vi "Get Scaled FP to PicBox.vi"(7 "仅可见区域":bool, 8 "错误输入（无错误）":errorcluster, 10 "图像参数":cluster{"图像深度":i32, "最大宽度":i32, "最大高度":i32}={"图像深度"=8, "最大宽度"=0, "最大高度"=0} {"图像深度" items=["1位、黑白"=1, "4位、16色"=4, "8位、256色"=8, "24位、真彩色"=24]}, 11 "VI Ref":refnum<vi>) -> (0 "错误输出":errorcluster, 3 "二维图片":picture)   [LabVIEW 2012, in "VIRef.lvlib"]
uses:
  VIRef.lvlib
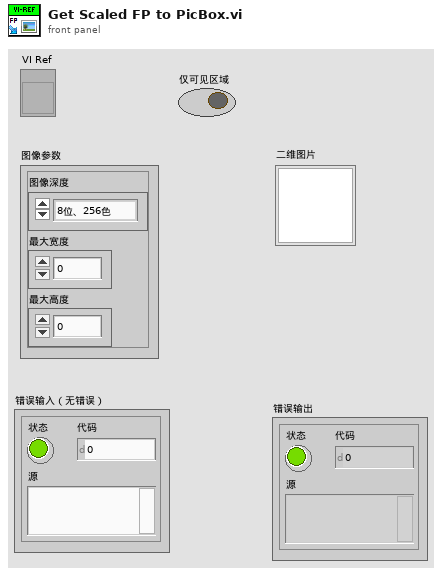
[diagram p1: front panel]
types:
  T1 = typedef "imagedata.ctl" = cluster{"image type":i32, "image depth":i32, "image":u8[], "mask":u8[], "colors":u32[], "Rectangle":cluster{"left":i16, "top":i16, "right":i16, "bottom":i16}}
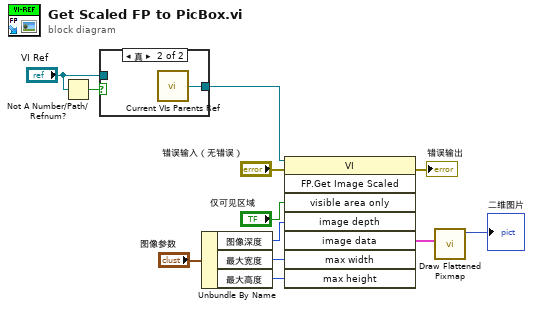
[diagram p0: block diagram]
diagram:
  n1 = Not A Number/Path/Refnum?(number/path/refnum="VI Ref") -> (NaN/Path/Refnum?=w12:bool)
  n2 = case shown="真" w12 {
    tunnel: [w13 w14] -> w10
    tunnel: "VI Ref" -> [w13 _]
    frame False {
    }
    frame True {
      n3 = call "Current VIs Parents Ref.vi"() -> ("Calling VI's Reference"=w14:refnum<vi>)  [unwired: 2 in]
    }
  }
  n4 = Unbundle By Name("图像参数") -> ("图像深度"=w7:i32, "最大宽度"=w6:i32, "最大高度"=w5:i32)
  n5 = invoke class="VI" method="FP.Get Image Scaled"(reference=w10, error in="错误输入（无错误）", "visible area only"="仅可见区域", "image depth"=w7, "max width"=w6, "max height"=w5) -> (error out=→"错误输出":errorcluster, "image data"=w2:T1)  [unwired: 2 in, 6 out]
  n6 = call <vilib>:"Draw Flattened Pixmap.vi"("image data"=w2) -> ("new picture"=→"二维图片":picture)  [unwired: 8 in]
